vi "MatrixSwitch.vi"(8 "error in (no error)":errorcluster, 10 "Action":T1(ring), 11 "LXIPXISwitching in":refnum<class "LXIPXISwitching.lvclass">) -> (0 "error out":errorcluster, 2 "Continue?":bool, 3 "LXIPXISwitching out":refnum<class "LXIPXISwitching.lvclass">)   [LabVIEW 2019, in "LXIPXISwitching.lvclass"]
uses:
  LXIPXISwitching.lvclass
  InstrumentSetup.vi
  InstrControl.lvclass
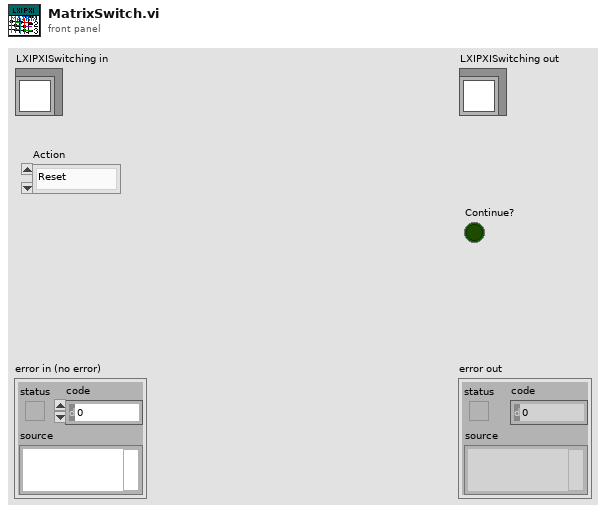
[diagram p1: front panel]
types:
  T1 = enum16{"Reset", "Ground", "Striptest Bias", "Striptest SMU", "Striptest LCR", "IV", "CV", "Interstrip Cap", "Interstrip Res"}
  T2 = cluster{"MUX":string, "Matrix":string, "Breadboard":string, "LXIPXI Switching":refnum<class "LXIPXISwitching.lvclass">, "MUX PN":string, "Matrix  PN":string, "Breadboard PN":string, "MUX ID":string, "Matrix ID":string, "Breadboard ID":string}
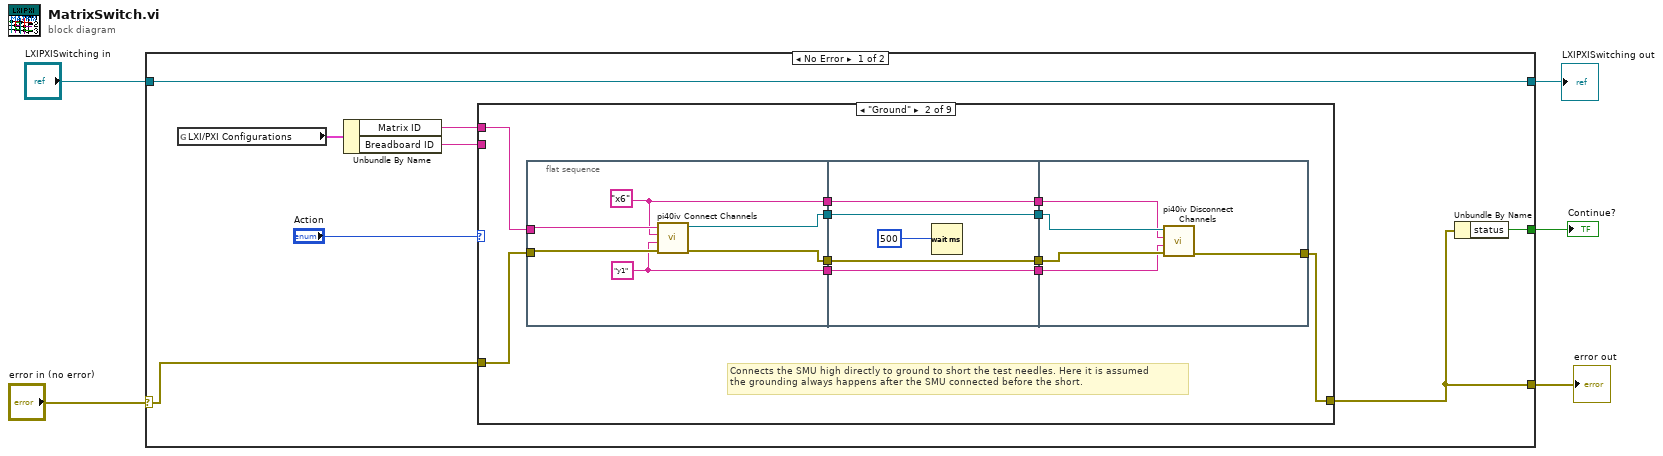
[diagram p0: block diagram]
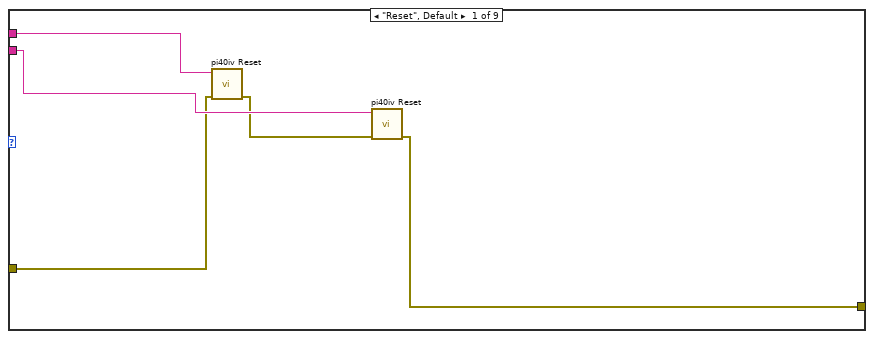
[diagram p2: hidden frame]
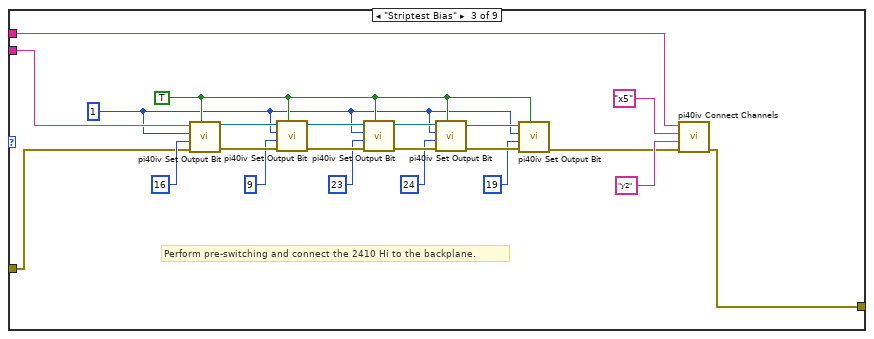
[diagram p3: hidden frame]
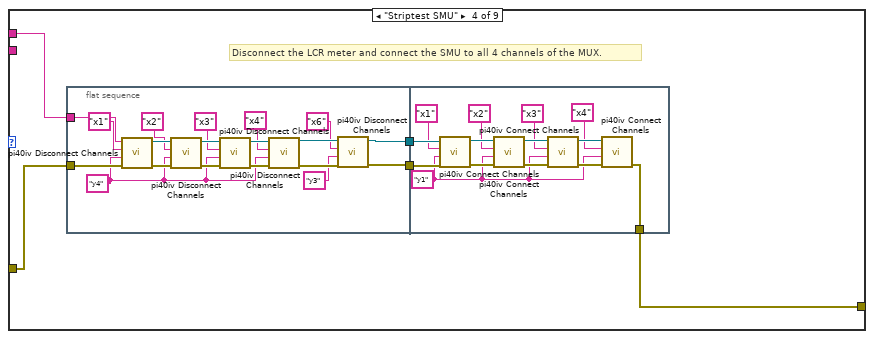
[diagram p4: hidden frame]
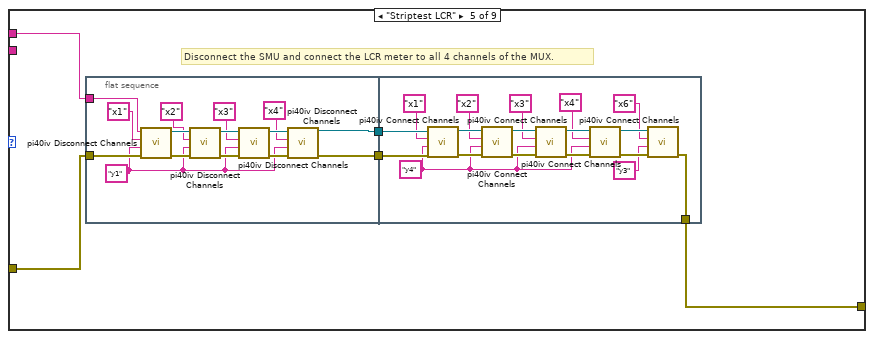
[diagram p5: hidden frame]
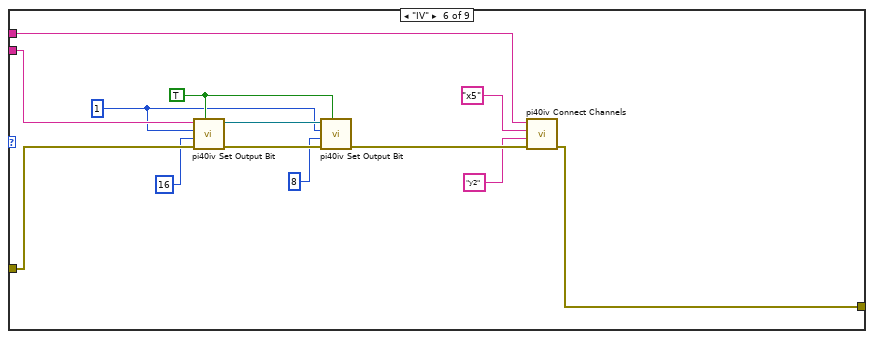
[diagram p6: hidden frame]
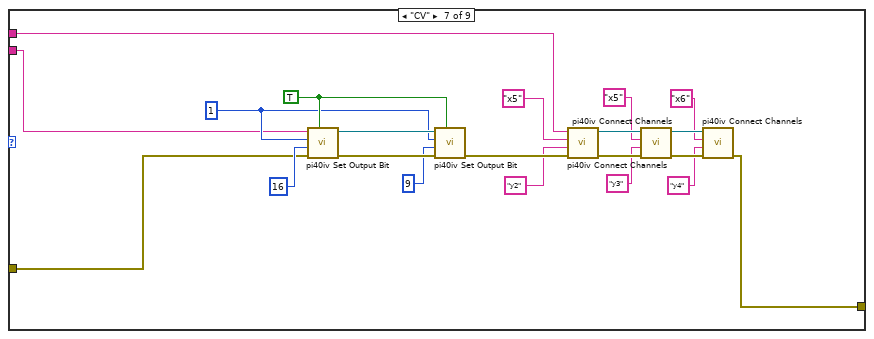
[diagram p7: hidden frame]
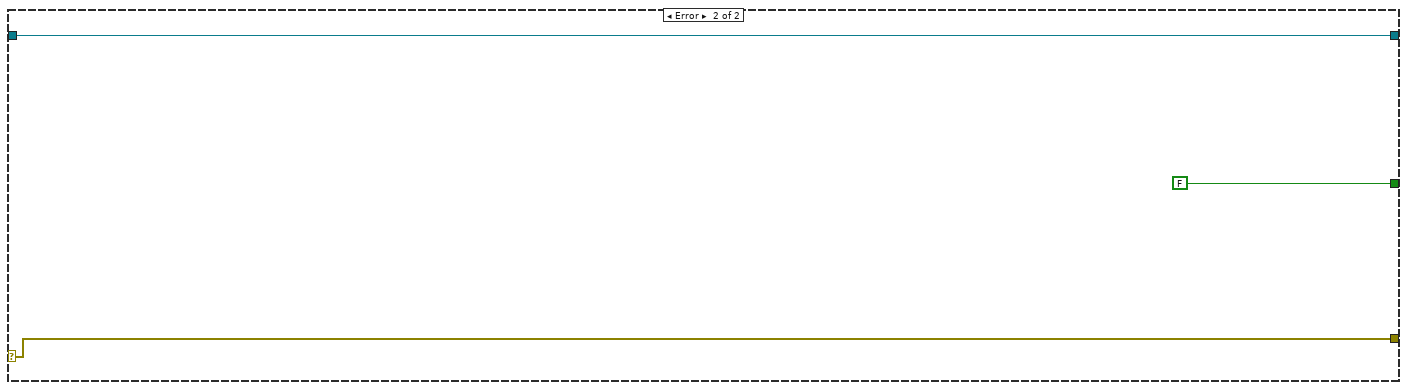
[diagram p10: hidden frame]
diagram:
  n1 = case shown="No Error" "error in (no error)" {
    selector: "error in (no error)" -> [w9 w182]
    tunnel: [w11 w180] -> w3
    tunnel: "LXIPXISwitching in" -> [w11 w180]
    tunnel: [w10 FALSE ("status")] -> w2
    tunnel: [w6 w182] -> w1
    frame No Error {
      n2 = global read "InstrumentSetup.vi" "LXI/PXI Configurations"() -> (w13:T2)
      n3 = Unbundle By Name(w13) -> ("Matrix ID"=w8:string, "Breadboard ID"=w7:string)
      n4 = case shown="\"Ground\"" "Action" {
        tunnel: w9 -> [w16 w28 w61 w70 w107 w152 w166 w178 w179]
        tunnel: w8 -> [w18 w29 w59 w72 w108 w155 w168 _ _]
        tunnel: w7 -> [w17 _ w60 _ _ w154 w167 _ _]
        tunnel: [w14 w24 w58 w68 w106 w149 w161 w178 w179] -> w6
        frame "Reset", Default {
          n5 = call <instrlib>:"pi40iv Reset.vi"("error in (no error)"=w16, "instrument handle"=w18) -> ("error out"=w15:errorcluster)  [unwired: 8 in, 1 out]
          n6 = call <instrlib>:"pi40iv Reset.vi"("error in (no error)"=w15, "instrument handle"=w17) -> ("error out"=w14:errorcluster)  [unwired: 8 in, 1 out]
        }
        frame "Ground" {
          # "Connects the SMU high directly to ground to short the test needles. Here it is assumed \nthe grounding always happens after the SMU connected before the short."
          n7 = flat-sequence {
            tunnel: w29 -> [w35]
            tunnel: w28 -> [w34]
            tunnel: [w32] -> w25
            tunnel: [w33] -> w23
            tunnel: [w31] -> w21
            tunnel: [w30] -> w19
            tunnel: [w39] -> w27
            tunnel: [w38] -> w26
            tunnel: w25 -> [w38]
            tunnel: w23 -> [w39]
            tunnel: [w37] -> w22
            tunnel: w21 -> [w37]
            tunnel: [w36] -> w20
            tunnel: w19 -> [w36]
            tunnel: w27 -> [w45]
            tunnel: w26 -> [w44]
            tunnel: [w43] -> w24
            tunnel: w22 -> [w42]
            tunnel: w20 -> [w41]
            frame #0 {
              w31 = "y1" ("channel 2")
              w30 = "x6" ("channel 1")
              n8 = call <instrlib>:"pi40iv Connect Channels.vi"("error in (no error)"=w34, "channel 2"=w31, "channel 1"=w30, "instrument handle"=w35) -> ("error out"=w32:errorcluster, "instrument handle out"=w33:refnum<k15>)  [unwired: 6 in]
            }
            frame #1 {
              n9 = Wait (ms)(milliseconds to wait=u32 500) -> ()  [unwired: 1 out]
            }
            frame #2 {
              n10 = call <instrlib>:"pi40iv Disconnect Channels.vi"("error in (no error)"=w44, "channel 2"=w42, "channel 1"=w41, "instrument handle"=w45) -> ("error out"=w43:errorcluster)  [unwired: 6 in, 1 out]
            }
          }
        }
        frame "Striptest Bias" {
          w47 = u32 1 ("output sub number")
          w49 = TRUE ("state")
          # "Perform pre-switching and connect the 2410 Hi to the backplane."
          n11 = call <instrlib>:"pi40iv Set Output Bit.vi"("state"=w49, "error in (no error)"=w61, "bit number"=u32 16, "output sub number"=w47, "instrument handle"=w60) -> ("error out"=w66:errorcluster, "instrument handle out"=w67:refnum<k15>)  [unwired: 5 in]
          n12 = call <instrlib>:"pi40iv Set Output Bit.vi"("state"=w49, "error in (no error)"=w66, "bit number"=u32 9, "output sub number"=w47, "instrument handle"=w67) -> ("error out"=w57:errorcluster, "instrument handle out"=w56:refnum<k15>)  [unwired: 5 in]
          n13 = call <instrlib>:"pi40iv Set Output Bit.vi"("state"=w49, "error in (no error)"=w57, "bit number"=u32 23, "output sub number"=w47, "instrument handle"=w56) -> ("error out"=w54:errorcluster, "instrument handle out"=w53:refnum<k15>)  [unwired: 5 in]
          n14 = call <instrlib>:"pi40iv Set Output Bit.vi"("state"=w49, "error in (no error)"=w54, "bit number"=u32 24, "output sub number"=w47, "instrument handle"=w53) -> ("error out"=w51:errorcluster, "instrument handle out"=w48:refnum<k15>)  [unwired: 5 in]
          n15 = call <instrlib>:"pi40iv Set Output Bit.vi"("state"=w49, "error in (no error)"=w51, "bit number"=u32 19, "output sub number"=w47, "instrument handle"=w48) -> ("error out"=w50:errorcluster)  [unwired: 5 in, 1 out]
          n16 = call <instrlib>:"pi40iv Connect Channels.vi"("error in (no error)"=w50, "channel 2"="y2", "channel 1"="x5", "instrument handle"=w59) -> ("error out"=w58:errorcluster)  [unwired: 6 in, 1 out]
        }
        frame "Striptest SMU" {
          # "Disconnect the LCR meter and connect the SMU to all 4 channels of the MUX."
          n17 = flat-sequence {
            tunnel: w72 -> [w91]
            tunnel: [w76] -> w71
            tunnel: w70 -> [w87]
            tunnel: [w75] -> w69
            tunnel: w71 -> [w105]
            tunnel: w69 -> [w101]
            tunnel: [w97] -> w68
            frame #0 {
              w79 = "y4" ("channel 2")
              n18 = call <instrlib>:"pi40iv Disconnect Channels.vi"("error in (no error)"=w87, "channel 2"=w79, "channel 1"="x1", "instrument handle"=w91) -> ("error out"=w86:errorcluster, "instrument handle out"=w90:refnum<k15>)  [unwired: 6 in]
              n19 = call <instrlib>:"pi40iv Disconnect Channels.vi"("error in (no error)"=w86, "channel 2"=w79, "channel 1"="x2", "instrument handle"=w90) -> ("error out"=w85:errorcluster, "instrument handle out"=w89:refnum<k15>)  [unwired: 6 in]
              n20 = call <instrlib>:"pi40iv Disconnect Channels.vi"("error in (no error)"=w85, "channel 2"=w79, "channel 1"="x3", "instrument handle"=w89) -> ("error out"=w84:errorcluster, "instrument handle out"=w88:refnum<k15>)  [unwired: 6 in]
              n21 = call <instrlib>:"pi40iv Disconnect Channels.vi"("error in (no error)"=w84, "channel 2"=w79, "channel 1"="x4", "instrument handle"=w88) -> ("error out"=w78:errorcluster, "instrument handle out"=w77:refnum<k15>)  [unwired: 6 in]
              n22 = call <instrlib>:"pi40iv Disconnect Channels.vi"("error in (no error)"=w78, "channel 2"="y3", "channel 1"="x6", "instrument handle"=w77) -> ("error out"=w75:errorcluster, "instrument handle out"=w76:refnum<k15>)  [unwired: 6 in]
            }
            frame #1 {
              w92 = "y1" ("channel 2")
              n23 = call <instrlib>:"pi40iv Connect Channels.vi"("error in (no error)"=w101, "channel 2"=w92, "channel 1"="x1", "instrument handle"=w105) -> ("error out"=w100:errorcluster, "instrument handle out"=w104:refnum<k15>)  [unwired: 6 in]
              n24 = call <instrlib>:"pi40iv Connect Channels.vi"("error in (no error)"=w100, "channel 2"=w92, "channel 1"="x2", "instrument handle"=w104) -> ("error out"=w99:errorcluster, "instrument handle out"=w103:refnum<k15>)  [unwired: 6 in]
              n25 = call <instrlib>:"pi40iv Connect Channels.vi"("error in (no error)"=w99, "channel 2"=w92, "channel 1"="x3", "instrument handle"=w103) -> ("error out"=w98:errorcluster, "instrument handle out"=w102:refnum<k15>)  [unwired: 6 in]
              n26 = call <instrlib>:"pi40iv Connect Channels.vi"("error in (no error)"=w98, "channel 2"=w92, "channel 1"="x4", "instrument handle"=w102) -> ("error out"=w97:errorcluster)  [unwired: 6 in, 1 out]
            }
          }
        }
        frame "Striptest LCR" {
          # "Disconnect the SMU and connect the LCR meter to all 4 channels of the MUX."
          n27 = flat-sequence {
            tunnel: w108 -> [w125]
            tunnel: [w112] -> w110
            tunnel: w107 -> [w121]
            tunnel: [w111] -> w109
            tunnel: w110 -> [w143]
            tunnel: w109 -> [w139]
            tunnel: [w126] -> w106
            frame #0 {
              w113 = "y1" ("channel 2")
              n28 = call <instrlib>:"pi40iv Disconnect Channels.vi"("error in (no error)"=w121, "channel 2"=w113, "channel 1"="x1", "instrument handle"=w125) -> ("error out"=w120:errorcluster, "instrument handle out"=w124:refnum<k15>)  [unwired: 6 in]
              n29 = call <instrlib>:"pi40iv Disconnect Channels.vi"("error in (no error)"=w120, "channel 2"=w113, "channel 1"="x2", "instrument handle"=w124) -> ("error out"=w119:errorcluster, "instrument handle out"=w123:refnum<k15>)  [unwired: 6 in]
              n30 = call <instrlib>:"pi40iv Disconnect Channels.vi"("error in (no error)"=w119, "channel 2"=w113, "channel 1"="x3", "instrument handle"=w123) -> ("error out"=w118:errorcluster, "instrument handle out"=w122:refnum<k15>)  [unwired: 6 in]
              n31 = call <instrlib>:"pi40iv Disconnect Channels.vi"("error in (no error)"=w118, "channel 2"=w113, "channel 1"="x4", "instrument handle"=w122) -> ("error out"=w111:errorcluster, "instrument handle out"=w112:refnum<k15>)  [unwired: 6 in]
            }
            frame #1 {
              w131 = "y4" ("channel 2")
              n32 = call <instrlib>:"pi40iv Connect Channels.vi"("error in (no error)"=w139, "channel 2"=w131, "channel 1"="x1", "instrument handle"=w143) -> ("error out"=w138:errorcluster, "instrument handle out"=w142:refnum<k15>)  [unwired: 6 in]
              n33 = call <instrlib>:"pi40iv Connect Channels.vi"("error in (no error)"=w138, "channel 2"=w131, "channel 1"="x2", "instrument handle"=w142) -> ("error out"=w137:errorcluster, "instrument handle out"=w141:refnum<k15>)  [unwired: 6 in]
              n34 = call <instrlib>:"pi40iv Connect Channels.vi"("error in (no error)"=w137, "channel 2"=w131, "channel 1"="x3", "instrument handle"=w141) -> ("error out"=w136:errorcluster, "instrument handle out"=w140:refnum<k15>)  [unwired: 6 in]
              n35 = call <instrlib>:"pi40iv Connect Channels.vi"("error in (no error)"=w136, "channel 2"=w131, "channel 1"="x4", "instrument handle"=w140) -> ("error out"=w129:errorcluster, "instrument handle out"=w130:refnum<k15>)  [unwired: 6 in]
              n36 = call <instrlib>:"pi40iv Connect Channels.vi"("error in (no error)"=w129, "channel 2"="y3", "channel 1"="x6", "instrument handle"=w130) -> ("error out"=w126:errorcluster)  [unwired: 6 in, 1 out]
            }
          }
        }
        frame "IV" {
          w144 = u32 1 ("output sub number")
          w156 = TRUE ("state")
          n37 = call <instrlib>:"pi40iv Set Output Bit.vi"("state"=w156, "error in (no error)"=w152, "bit number"=u32 16, "output sub number"=w144, "instrument handle"=w154) -> ("error out"=w151:errorcluster, "instrument handle out"=w153:refnum<k15>)  [unwired: 5 in]
          n38 = call <instrlib>:"pi40iv Set Output Bit.vi"("state"=w156, "error in (no error)"=w151, "bit number"=u32 8, "output sub number"=w144, "instrument handle"=w153) -> ("error out"=w150:errorcluster)  [unwired: 5 in, 1 out]
          n39 = call <instrlib>:"pi40iv Connect Channels.vi"("error in (no error)"=w150, "channel 2"="y2", "channel 1"="x5", "instrument handle"=w155) -> ("error out"=w149:errorcluster)  [unwired: 6 in, 1 out]
        }
        frame "CV" {
          w169 = u32 1 ("output sub number")
          w177 = TRUE ("state")
          n40 = call <instrlib>:"pi40iv Set Output Bit.vi"("state"=w177, "error in (no error)"=w166, "bit number"=u32 16, "output sub number"=w169, "instrument handle"=w167) -> ("error out"=w175:errorcluster, "instrument handle out"=w176:refnum<k15>)  [unwired: 5 in]
          n41 = call <instrlib>:"pi40iv Set Output Bit.vi"("state"=w177, "error in (no error)"=w175, "bit number"=u32 9, "output sub number"=w169, "instrument handle"=w176) -> ("error out"=w174:errorcluster)  [unwired: 5 in, 1 out]
          n42 = call <instrlib>:"pi40iv Connect Channels.vi"("error in (no error)"=w174, "channel 2"="y2", "channel 1"="x5", "instrument handle"=w168) -> ("error out"=w163:errorcluster, "instrument handle out"=w165:refnum<k15>)  [unwired: 6 in]
          n43 = call <instrlib>:"pi40iv Connect Channels.vi"("error in (no error)"=w163, "channel 2"="y3", "channel 1"="x5", "instrument handle"=w165) -> ("error out"=w162:errorcluster, "instrument handle out"=w164:refnum<k15>)  [unwired: 6 in]
          n44 = call <instrlib>:"pi40iv Connect Channels.vi"("error in (no error)"=w162, "channel 2"="y4", "channel 1"="x6", "instrument handle"=w164) -> ("error out"=w161:errorcluster)  [unwired: 6 in, 1 out]
        }
        frame "Interstrip Cap" {
          # "To be done..."
        }
        frame "Interstrip Res" {
          # "To be done..."
        }
      }
      n45 = Unbundle By Name(w6) -> ("status"=w10:bool)
    }
    frame Error {
    }
  }
  "error out" <- w1
  "LXIPXISwitching out" <- w3
  "Continue?" <- w2
